vi "Error Popup 1523.vi"(4 "Error In":errorcluster, 7 "Error":string) -> (0 "Error Out":errorcluster)   [LabVIEW 2015]
panel:
  in  "OK Button":bool
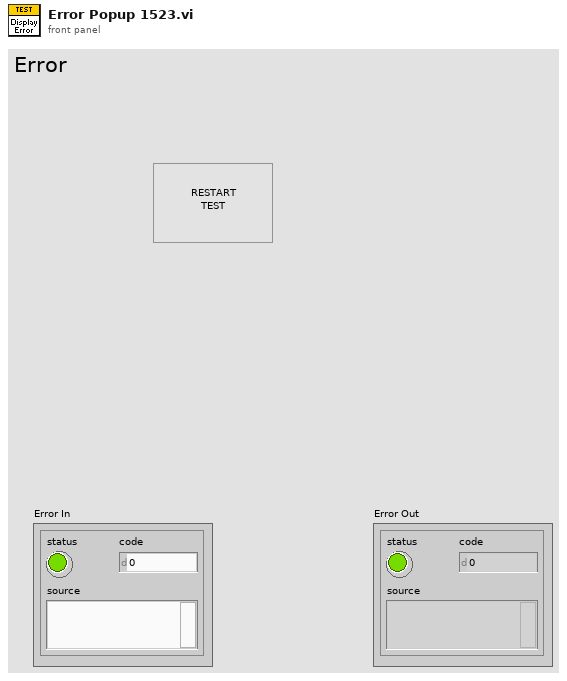
[diagram p1: front panel]
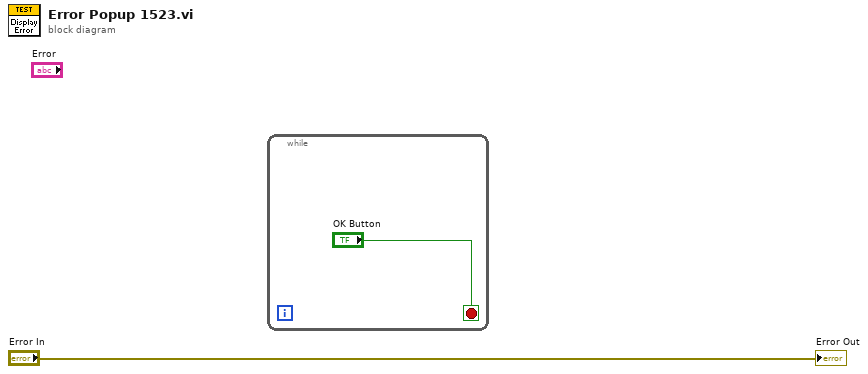
[diagram p0: block diagram]
diagram:
  n1 = while {
    stop <- "OK Button" stop-if-true
  }
  "Error Out" <- "Error In"
